vi "getUnitsByChannelName.vi"(8 "error in (no error)":errorcluster, 10 "channel_name":string, 11 "ChannelArray in":refnum<class "ChannelArray.lvclass">) -> (0 "error out":errorcluster, 2 "units":string, 3 "ChannelArray out":refnum<class "ChannelArray.lvclass">)   [LabVIEW 2009, in "Tools.lvlib" / "DatabaseHelpers.lvlib" / "ChannelArray.lvclass"]
uses:
  ChannelArray.lvclass
  Channel/Channel.lvclass
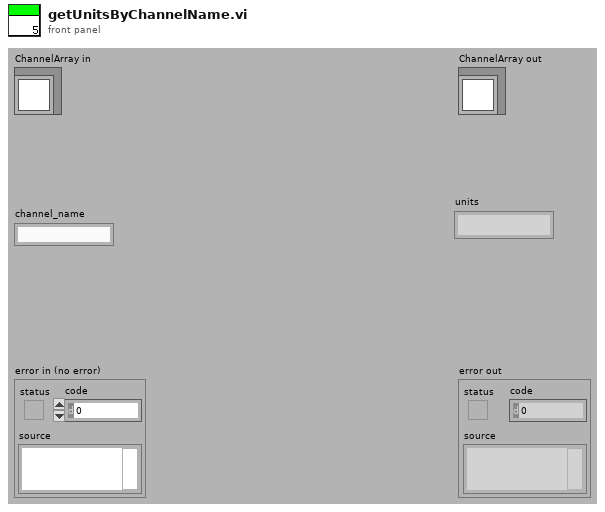
[diagram p1: front panel]
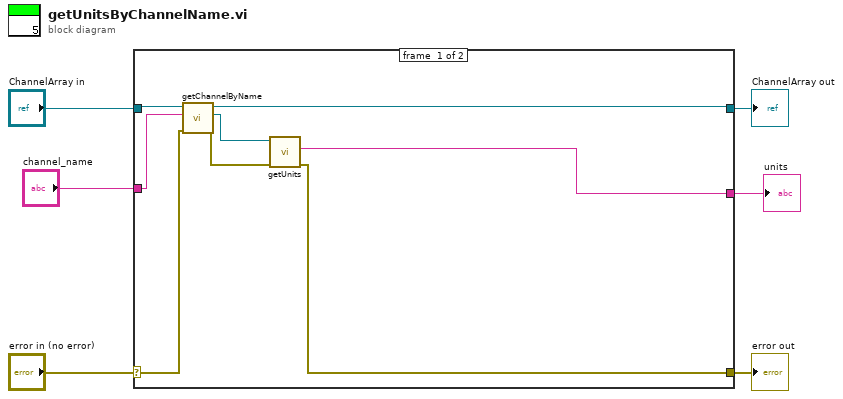
[diagram p0: block diagram]
diagram:
  n1 = case shown="No Error" "error in (no error)" {
    selector: "error in (no error)" -> [w10 w16]
    tunnel: [w9 w16] -> w5
    tunnel: [w13 w15] -> w3
    tunnel: "ChannelArray in" -> [w14 w15]
    tunnel: [w8 _] -> w2
    tunnel: "channel_name" -> [w7 _]
    frame #0 {
      n2 = call-dynamic "getChannelByName.vi"("error in (no error)"=w10, "channel_name"=w7, "ChannelArray in"=w14) -> ("error out"=w11:errorcluster, "Channel"=w12:refnum<class "Channel.lvclass">, "ChannelArray out"=w13:refnum<class "ChannelArray.lvclass">)  [unwired: 5 in, 1 out]
      n3 = call-dynamic "getUnits.vi"("error in (no error)"=w11, "Channel.lvclass in"=w12) -> ("error out"=w9:errorcluster, "units"=w8:string)  [unwired: 7 in, 1 out]
    }
    frame #1 {
    }
  }
  "error out" <- w5
  "ChannelArray out" <- w3
  "units" <- w2
